vi "Configure Module.vi"(8 "error in (no error)":errorcluster, 10 "IOV ref in":refnum<k21>, 11 "Module Template in":refnum<class "9209.lvclass">) -> (0 "error out":errorcluster, 2 "IOV ref out":refnum<k21>, 3 "Module Template out":refnum<class "9209.lvclass">)   [LabVIEW 2019, in "Modules.lvlib" / "9209.lvclass"]
uses:
  9209.lvclass
  9209.lvclass/9209.ctl
  <resource>/objmgr/cRIO.rc
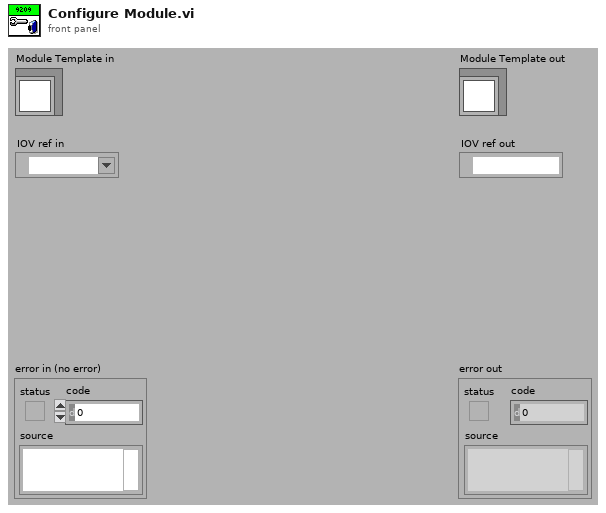
[diagram p1: front panel]
types:
  T1 = typedef "Modules.lvlib/9209.lvclass/Channel Settings.ctl" = T2[]
  T2 = typedef "Modules.lvlib/9209.lvclass/Terminal mode.ctl" = enum16{"RSE", "DIFF"}
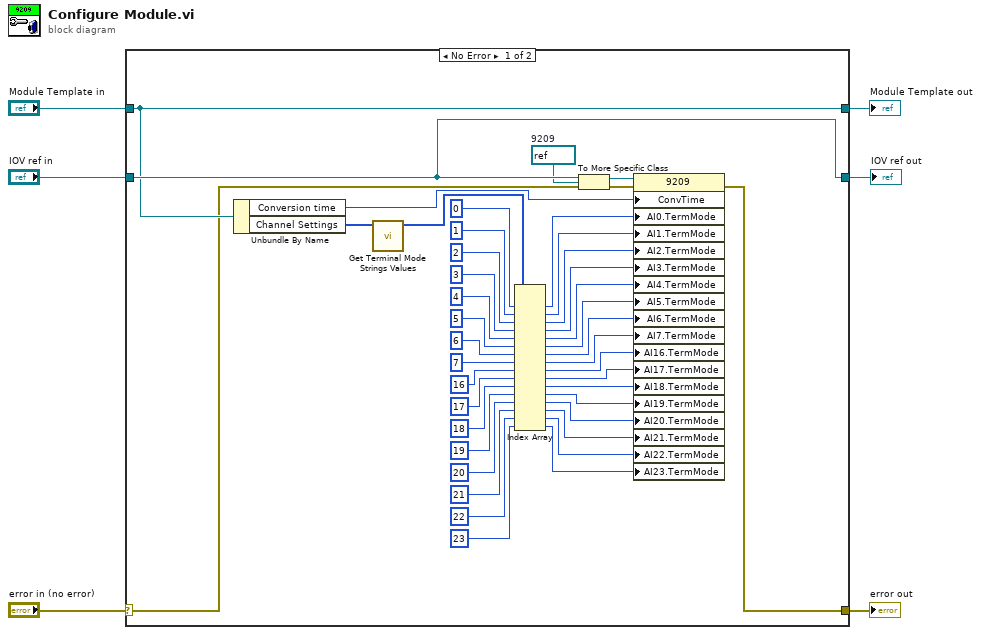
[diagram p0: block diagram]
diagram:
  n1 = case shown="No Error" "error in (no error)" {
    selector: "error in (no error)" -> [w44 w51]
    tunnel: [w48 w51] -> w5
    tunnel: [w45 w50] -> w3
    tunnel: "Module Template in" -> [w45 w50]
    tunnel: "IOV ref in" -> [w47 w49]
    tunnel: [w47 w49] -> w1
    frame No Error {
      w43 = refnum<k21> refnum  # 9209
      n2 = Unbundle By Name(w45) -> ("Conversion time"=w46:u32, "Channel Settings"=w8:T1)
      n3 = call "Get Terminal Mode Strings Values.vi"("Terminal Mode Display Values"=w8) -> ("Terminal Mode RSI Values"=w7:u32[])  [unwired: 10 in]
      n4 = Index Array(array=w7, index #1=0 ("index"), index #2=1 ("index"), index #3=2 ("index"), index #4=3 ("index"), index #5=4 ("index"), index #6=5 ("index"), index #7=6 ("index"), index #8=7 ("index"), index #9=16 ("index"), index #10=17 ("index"), index #11=18 ("index"), index #12=19 ("index"), index #13=20 ("index"), index #14=21 ("index"), index #15=22 ("index"), index #16=23 ("index")) -> (element #1=w24:u32, element #2=w23:u32, element #3=w22:u32, element #4=w21:u32, element #5=w20:u32, element #6=w19:u32, element #7=w18:u32, element #8=w17:u32, element #9=w16:u32, element #10=w15:u32, element #11=w14:u32, element #12=w13:u32, element #13=w12:u32, element #14=w11:u32, element #15=w9:u32, element #16=w10:u32)
      n5 = To More Specific Class(target class=w43, reference=w47, error in=w44) -> (specific class reference=w42:refnum<k21>, error out=w41:errorcluster)
      n6 = property class="9209"(reference=w42, error in=w41, "ConvTime"=w46, "AI0.TermMode"=w24, "AI1.TermMode"=w23, "AI2.TermMode"=w22, "AI3.TermMode"=w21, "AI4.TermMode"=w20, "AI5.TermMode"=w19, "AI6.TermMode"=w18, "AI7.TermMode"=w17, "AI16.TermMode"=w16, "AI17.TermMode"=w15, "AI18.TermMode"=w14, "AI19.TermMode"=w13, "AI20.TermMode"=w12, "AI21.TermMode"=w11, "AI22.TermMode"=w9, "AI23.TermMode"=w10) -> (error out=w48:errorcluster)  [unwired: 1 out]
    }
    frame Error {
    }
  }
  "error out" <- w5
  "Module Template out" <- w3
  "IOV ref out" <- w1
